vi "FunkcjonalnaZmiennaGlobalna.vi"(2 "Wejœcie":dbl, 3 "Stan":T1) -> (0 "Wyjœcie":dbl)   [LabVIEW 2024]
uses:
  FZG.ctl
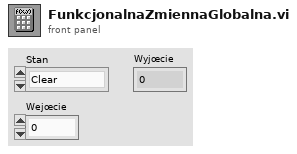
[diagram p1: front panel]
types:
  T1 = typedef "FZG.ctl" = enum16{"Clear", "AddElement", "SubElement", "MulElement", "DivElement", "PowElement"}
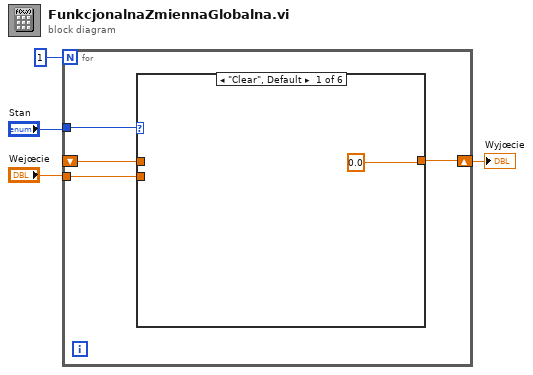
[diagram p0: block diagram]
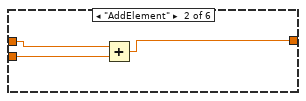
[diagram p2: hidden frame]
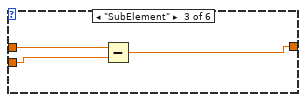
[diagram p3: hidden frame]
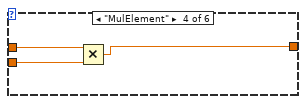
[diagram p4: hidden frame]
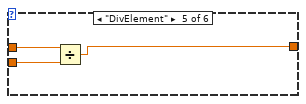
[diagram p5: hidden frame]
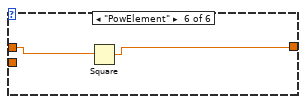
[diagram p6: hidden frame]
diagram:
  n1 = for {
    N: 1 -> [_]
    shift-right: [w7] -> w1
    shift-left: _ -> [w6]
    tunnel: "Stan" -> [w8]
    tunnel: "Wejœcie" -> [w5]
    n2 = case shown="\"Clear\", Default" w8 {
      tunnel: [0.0 w10 w13 w16 w19 w22] -> w7
      tunnel: w6 -> [_ w12 w15 w18 w21 w23]
      tunnel: w5 -> [_ w11 w14 w17 w20 _]
      frame "Clear", Default {
      }
      frame "AddElement" {
        n3 = Add(x=w12, y=w11) -> (x+y=w10:dbl)
      }
      frame "SubElement" {
        n4 = Subtract(x=w15, y=w14) -> (x-y=w13:dbl)
      }
      frame "MulElement" {
        n5 = Multiply(x=w18, y=w17) -> (x*y=w16:dbl)
      }
      frame "DivElement" {
        n6 = Divide(x=w21, y=w20) -> (x/y=w19:dbl)
      }
      frame "PowElement" {
        n7 = Square(x=w23) -> (x^2=w22:dbl)
      }
    }
  }
  "Wyjœcie" <- w1
